vi "字符补长.vi"(1 "in":string) -> (0 "out":string)   [LabVIEW 2015, in "AN97005N.lvlib"]
uses:
  AN97005N.lvlib
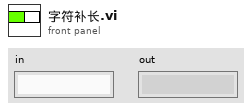
[diagram p1: front panel]
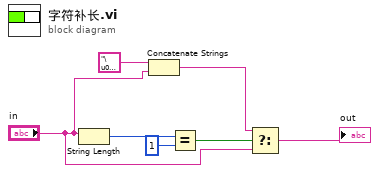
[diagram p0: block diagram]
diagram:
  n1 = String Length(string="in") -> (length=w7:i32)
  n2 = Concatenate Strings("\u0000", "in") -> (w3:string)
  n3 = Equal?(x=w7, y=1) -> (x = y?=w5:bool)
  n4 = Select(t=w3, s=w5, f="in") -> (s? t:f=→"out":string)
